vi "PTestbed_Cycling.vi"() -> ()   [LabVIEW 2020]
uses:
  Drivers-IT-M3400/IT-M3400.lvlib
panel:
  out "DAQ error out":errorcluster[](array[cluster])
  out "PS error out":errorcluster[](array[cluster])
  in  "Current Cutoff":dbl
  in  "Charge filepath":path
  in  "Discharge filepath":path
  in  "Testname":string
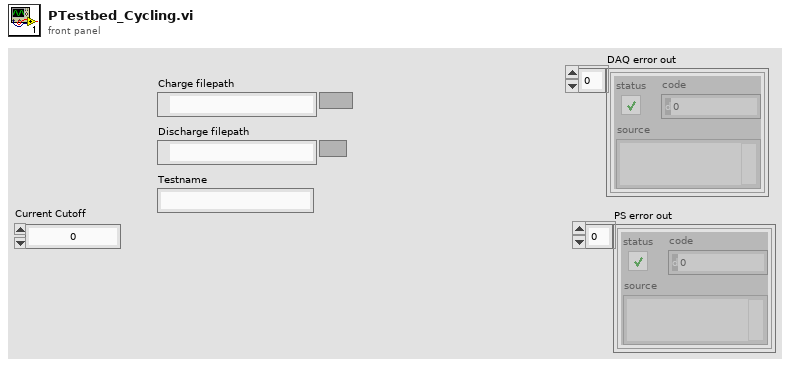
[diagram p1: front panel]
types:
  T1 = enum16{"Battery 1", "Battery 2", "Battery 3", "Battery 1&2", "Battery 1&3", "Battery 2&3", "Battery 1&2&3"}
  T2 = enum16{"\"30Q\"", "\"40T\"", "\"2P30Q\"", "\"3P30Q\"", "\"Nissan Leaf\"", ""}
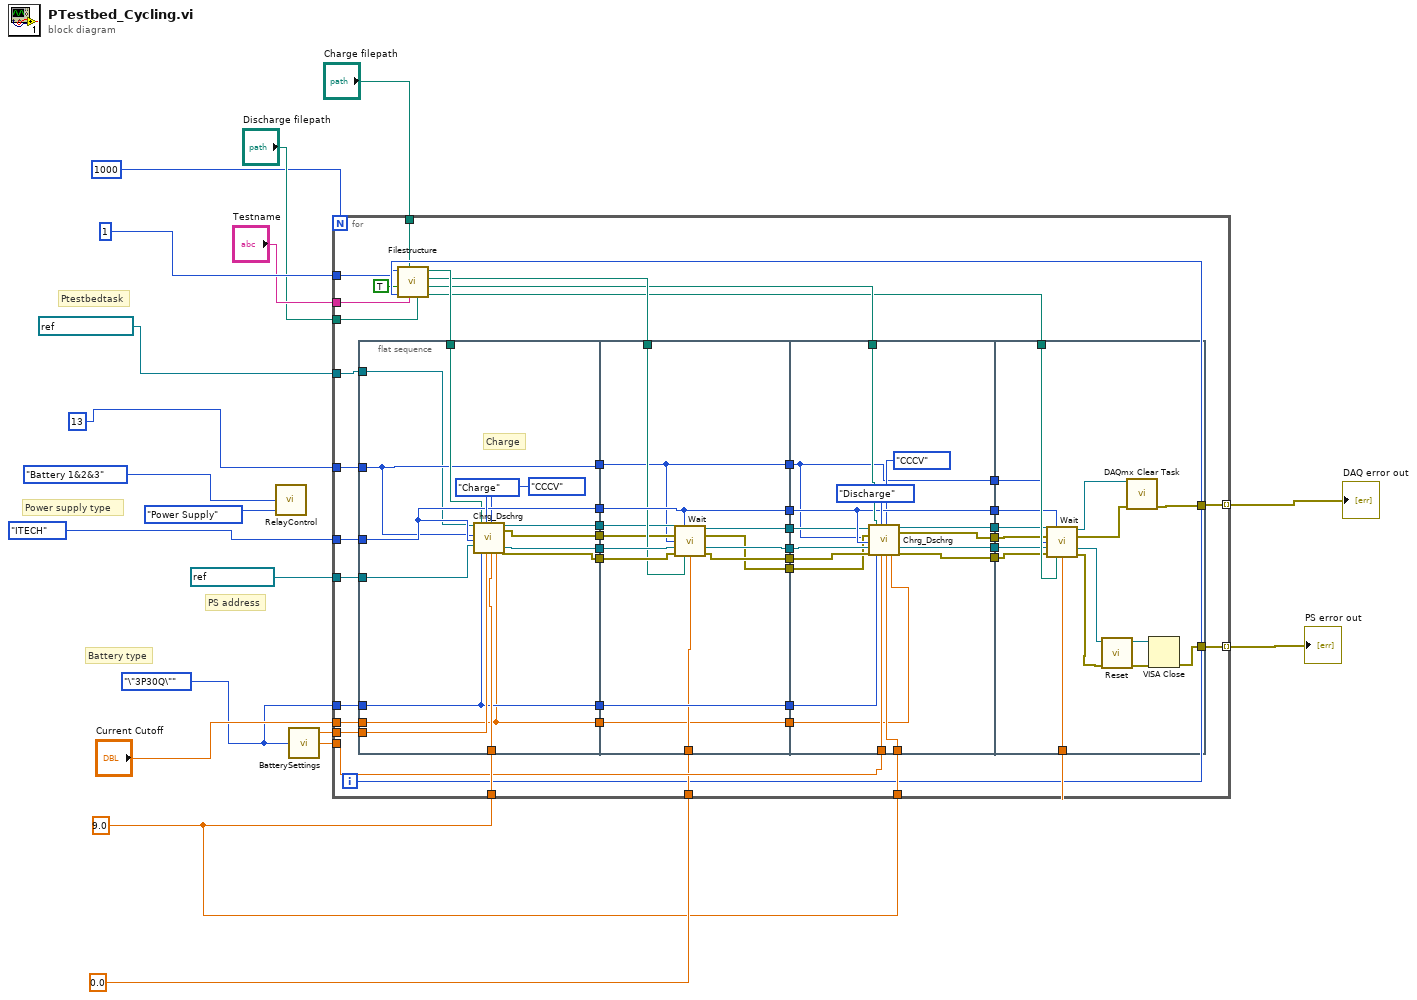
[diagram p0: block diagram]
diagram:
  w1 = 9.0 ("Charge Current Setpoint")
  w3 = T2."\"3P30Q\"" ("Battery Type")
  # "Battery type"
  # "PS address"
  # "Power supply type"
  # "Ptestbedtask"
  n1 = call "RelayControl.vi"("NHR or Battery Analyzer"=enum16{"Battery Analyzer", "Power Supply"}."Power Supply", "Battery Select"=T1."Battery 1&2&3") -> ()  [unwired: 3 in]
  n2 = call "BatterySettings.vi"("Battery Type"=w3) -> ("Min Voltage (V)"=w18:dbl, "Max Voltage (V)"=w19:dbl)  [unwired: 2 in, 1 out]
  n3 = for {
    N: 1000 ("Number of Cycles") -> [_]
    tunnel: 13 ("#DAQ outputs (1-13)") -> [w51]
    tunnel: enum16{"NHR", "ITECH"}."ITECH" ("PS type") -> [w50]
    tunnel: w19 -> [w49]
    tunnel: w3 -> [w48]
    tunnel: w1 -> [w47]
    tunnel: w18 -> [w46]
    tunnel: w1 -> [w45]
    tunnel: 0.0 ("Wait time") -> [w40]
    tunnel: 1 ("Starting Cycle") -> [w38]
    tunnel: "Testname" -> [w36]
    tunnel: "Discharge filepath" -> [w35]
    tunnel: "Charge filepath" -> [w34]
    tunnel: "Current Cutoff" -> [w33]
    tunnel: [w23] -> w7 mode=indexing
    tunnel: [w22] -> w6 mode=indexing
    tunnel: refnum<k21> "PTesbedTask" ("Data Task in") -> [w21]
    tunnel: refnum<visa-resource-name> "ITECH-PS3" ("PS Visa Out") -> [w20]
    i -> [w39]
    n4 = flat-sequence {
      tunnel: w21 -> [w70]
      tunnel: w51 -> [w71]
      tunnel: w50 -> [w74]
      tunnel: w48 -> [w73]
      tunnel: w49 -> [w78]
      tunnel: w47 -> [w77]
      tunnel: [w76] -> w64
      tunnel: [w75] -> w63
      tunnel: [w74] -> w62
      tunnel: [w71] -> w61
      tunnel: [w73] -> w60
      tunnel: w44 -> [w72]
      tunnel: w33 -> [w68]
      tunnel: [w68] -> w32
      tunnel: [w67] -> w30
      tunnel: [w66] -> w29
      tunnel: w20 -> [w65]
      tunnel: w64 -> [w93]
      tunnel: w63 -> [w92]
      tunnel: w62 -> [w89]
      tunnel: [w91] -> w59
      tunnel: [w90] -> w58
      tunnel: w61 -> [w80]
      tunnel: [w80] -> w57
      tunnel: [w89] -> w56
      tunnel: w60 -> [w88]
      tunnel: [w88] -> w55
      tunnel: w43 -> [w87]
      tunnel: w40 -> [w86]
      tunnel: w32 -> [w85]
      tunnel: [w85] -> w31
      tunnel: w30 -> [w84]
      tunnel: w29 -> [w83]
      tunnel: [w82] -> w28
      tunnel: [w81] -> w27
      tunnel: w59 -> [w110]
      tunnel: w58 -> [w109]
      tunnel: w57 -> [w94]
      tunnel: w56 -> [w101]
      tunnel: w55 -> [w108]
      tunnel: w46 -> [w107]
      tunnel: w45 -> [w106]
      tunnel: w42 -> [w104]
      tunnel: [w103] -> w54
      tunnel: [w102] -> w53
      tunnel: [w101] -> w52
      tunnel: w31 -> [w99]
      tunnel: w28 -> [w98]
      tunnel: w27 -> [w97]
      tunnel: [w96] -> w26
      tunnel: [w95] -> w25
      tunnel: [w94] -> w24
      tunnel: w41 -> [w126]
      tunnel: w54 -> [w125]
      tunnel: w53 -> [w124]
      tunnel: w40 -> [w123]
      tunnel: w52 -> [w122]
      tunnel: [w115] -> w23
      tunnel: w26 -> [w121]
      tunnel: w25 -> [w120]
      tunnel: [w116] -> w22
      tunnel: w24 -> [w119]
      frame #0 {
        # "Charge"
        n5 = call "Chrg_Dschrg.vi"("Data Task in"=w70, "#DAQ outputs (1-13)"=w71, "PS type"=w74, "PS VISA in"=w65, "DischargeCyclePath"=w72, "Battery Type"=w73, "Charge/discharge"=enum8{"Charge", "Discharge"}."Charge", "Charge/Discharge Voltage Setpoint"=w78, "CC or CCCV"=enum16{"CC", "CCCV"}."CCCV", "Current Setpoint"=w77, "Current Cutoff"=w68) -> ("data task out"=w67:refnum<k21>, "data task error out"=w66:errorcluster, "PS VIS resource name out"=w76:refnum<visa-resource-name>, "PS error out"=w75:errorcluster)  [unwired: 5 in]
      }
      frame #1 {
        n6 = call "Wait.vi"("Data Task in"=w84, "PS type"=w89, "data task error in"=w83, "#DAQ outputs (1-13)"=w80, "PS VISA in"=w93, "PS error in"=w92, "Wait Filepath"=w87, "Wait time"=w86) -> ("data task out"=w82:refnum<k21>, "data task error out"=w81:errorcluster, "PS Visa Out"=w91:refnum<visa-resource-name>, "PS error out"=w90:errorcluster)  [unwired: 4 in]
      }
      frame #2 {
        n7 = call "Chrg_Dschrg.vi"("Data Task in"=w98, "data task error in"=w97, "#DAQ outputs (1-13)"=w94, "PS type"=w101, "PS VISA in"=w110, "PS error in"=w109, "DischargeCyclePath"=w104, "Battery Type"=w108, "Charge/discharge"=enum8{"Charge", "Discharge"}."Discharge", "Charge/Discharge Voltage Setpoint"=w107, "CC or CCCV"=enum16{"CC", "CCCV"}."CCCV", "Current Setpoint"=w106, "Current Cutoff"=w99) -> ("data task out"=w96:refnum<k21>, "data task error out"=w95:errorcluster, "PS VIS resource name out"=w103:refnum<visa-resource-name>, "PS error out"=w102:errorcluster)  [unwired: 3 in]
      }
      frame #3 {
        n8 = call "Wait.vi"("Data Task in"=w121, "PS type"=w122, "data task error in"=w120, "#DAQ outputs (1-13)"=w119, "PS VISA in"=w125, "PS error in"=w124, "Wait Filepath"=w126, "Wait time"=w123) -> ("data task out"=w118:refnum<k21>, "data task error out"=w117:errorcluster, "PS Visa Out"=w114:refnum<visa-resource-name>, "PS error out"=w113:errorcluster)  [unwired: 4 in]
        n9 = call "Reset.vi"("error in"=w113, "VISA resource name"=w114) -> ("error out"=w112:errorcluster, "VISA resource name out"=w111:refnum<visa-resource-name>)  [unwired: 8 in]
        n10 = call <vilib>:"DAQmx Clear Task.vi"("task in"=w118, "error in"=w117) -> ("error out"=w116:errorcluster)  [unwired: 13 in]
        n11 = VISA Close(VISA resource name=w111, error in (no error)=w112) -> (error out=w115:errorcluster)
      }
    }
    n12 = call "Filestructure.vi"("Discharge filepath"=w35, "Batteryname"=w36, "Charge filepath"=w34, "For loop i"=w39, "In for loop"=TRUE, "Starting Cycle"=w38) -> ("DischargeWaitPath"=w41:path, "DischargeCyclePath"=w42:path, "ChargeWaitPath"=w43:path, "ChargeCyclePath"=w44:path)  [unwired: 1 in, 1 out]
  }
  "PS error out" <- w7
  "DAQ error out" <- w6
